vi "onPrevious.vi"(8 "error in (no error)":errorcluster, 10 "Player In":refnum<class "Player.lvclass">, 11 "LockedState in":refnum<class "LockedState.lvclass">) -> (0 "error out":errorcluster, 1 "String":string, 2 "Player Out":refnum<class "Player.lvclass">, 3 "LockedState out":refnum<class "LockedState.lvclass">)   [LabVIEW 2018, in "LockedState.lvclass"]
uses:
  LockedState.lvclass
  Player Class/Player.lvclass
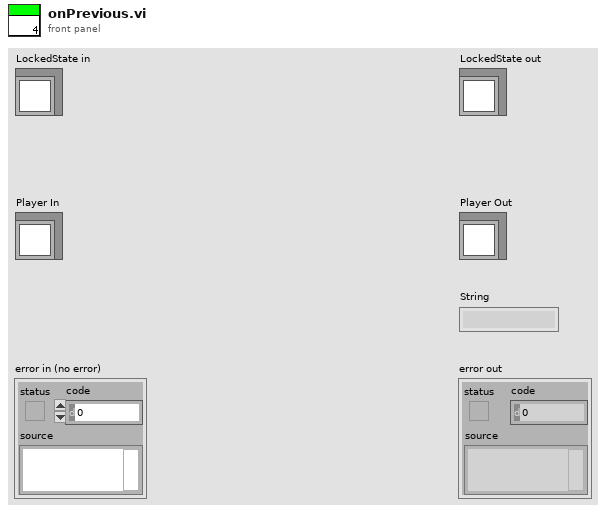
[diagram p1: front panel]
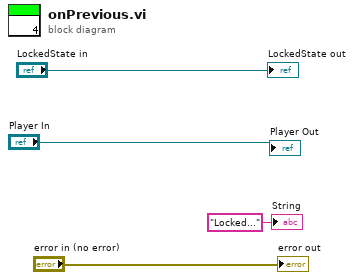
[diagram p0: block diagram]
diagram:
  "error out" <- "error in (no error)"
  "LockedState out" <- "LockedState in"
  "String" <- "Locked..." ("String")
  "Player Out" <- "Player In"
